vi "Verwaltung Betriebsstundenzaehler.vi"(8 "Zeitstempel Syslog":timestamp, 10 "Zeitstempel FT-IR":timestamp, 11 "Zeitstempel BMP":timestamp) -> (0 "Zeitstempel Syslog":timestamp, 2 "Zeitstempel FT-IR":timestamp, 3 "Zeitstempel BMP":timestamp)   [LabVIEW 2020, in "Betriebsstundenzaehler.lvlib"]
uses:
  Betriebsstundenzaehler.lvlib
  Allgemein/FGV Zustaende Aktionen.ctl
  FGV BSZ Aktionen.ctl
  Konfig-Dateien/Aktionen Konfig.ctl
  Regler/Druckregler/Aktionen Interne Werte.ctl
  SysLog/SysLog Interface cRIO.ctl
  Konfig-Dateien/Konfig-Dateien.lvlib
  Regler/Druckregler/Druckregler.lvlib
  Allgemein/Allgemein.lvlib
  SysLog/SysLog_cRIO.lvlib
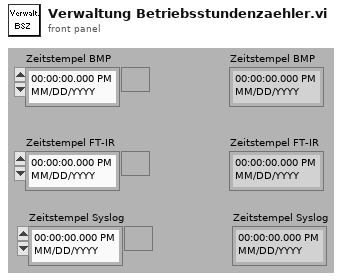
[diagram p1: front panel]
types:
  T1 = typedef "Allgemein.lvlib/FGV Zustaende Aktionen.ctl" = enum16{"lesen", "Zustand PC", "Zustand cRIO", "Bildnummer", "Samplepoint", "Sysloglevel"}
  T2 = typedef "Betriebsstundenzaehler.lvlib/FGV BSZ Aktionen.ctl" = enum16{"Lesen", "Initialisieren", "Starten Pumpe", "Zählen Pumpe", "Starten FT-IR", "Zählen FT-IR"}
  T3 = typedef "Regler.lvlib/Druckregler.lvlib/Aktionen Interne Werte.ctl" = enum16{"lesen", "FT-IR", "Ausgang", "Pumpe", "laden", "speichern", "Änderung?", "Druck Kalter Block", "Dichtheitstest"}
  T4 = typedef "Konfig-Dateien.lvlib/Aktionen Konfig.ctl" = enum16{"lesen", "laden", "speichern  System.ini", "speichern Anlagengrenzw.", "speichern PID + Sonstige", "speichern BSZ BMP", "speichern BSZ FT-IR", "speichern Stickstoff Bef.", "speichern Ext. Stickstoff Bef.", "speichern CAN_Konfig"}
  T5 = typedef "SysLog_cRIO.lvlib/SysLog Interface cRIO.ctl" = cluster{"FehlermeldungsCode":i32, "ErfolgsmeldungsCode":i32, "ParameterListenString":string, "intern":bool}
  T6 = typedef "Funktionstasten.lvlib/Zustaende.ctl" = enum16{"Standby", "Pause", "Eco", "Messen", "Kalibrieren", "Spülen Filter", "Spülen Leitung", "Umgebungsluft", "0-Gas", "Cal-Gas", "CG zu PNS", "-------------", "Init 1", "Init 2", "Init 3", "Init 4", "Messen vorbereiten", "Messen durchführen", "Exit"}
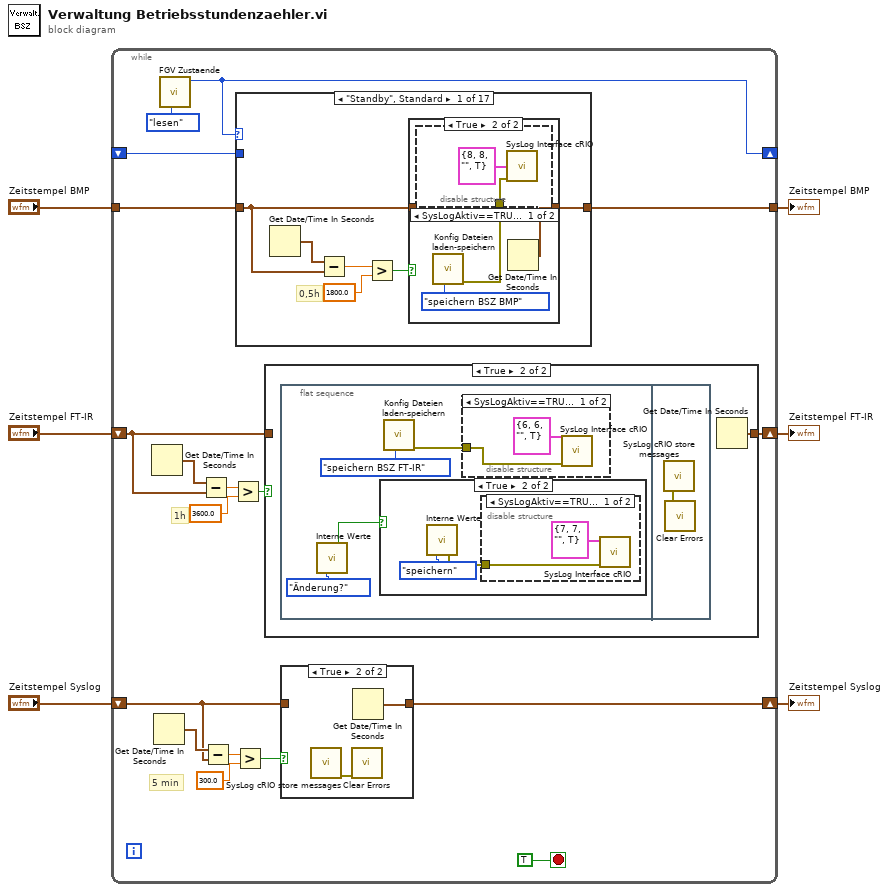
[diagram p0: block diagram]
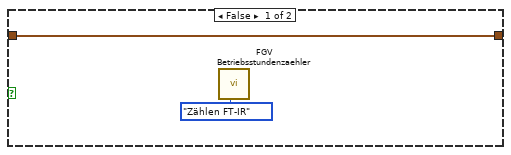
[diagram p3: hidden frame]
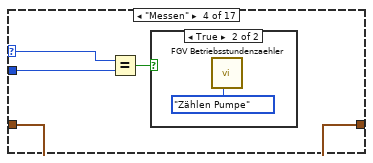
[diagram p11: hidden frame]
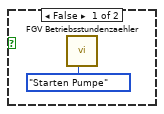
[diagram p12: hidden frame]
diagram:
  n1 = while {
    shift-right: [w13] -> _
    shift-left: _ -> [w23]
    tunnel: "Zeitstempel BMP" -> [w22]
    tunnel: [w21] -> w5
    shift-right: [w15] -> w3
    shift-left: "Zeitstempel FT-IR" -> [w16]
    shift-right: [w7] -> w1
    shift-left: "Zeitstempel Syslog" -> [w8]
    stop <- TRUE stop-if-true
    # "5 min"
    # "1h"
    n2 = Get Date/Time In Seconds() -> (seconds since 1Jan1904=w17:timestamp)
    n3 = Get Date/Time In Seconds() -> (seconds since 1Jan1904=w12:timestamp)
    n4 = call "FGV Zustaende.vi"("Aktionen"=FGV_Zustaende_Aktionen."lesen") -> ("Zustand PC"=w13:T6)  [unwired: 6 in, 4 out]
    n5 = Subtract(x=w17, y=w16) -> (x-y=w18:dbl)
    n6 = Subtract(x=w12, y=w8) -> (x-y=w11:dbl)
    n7 = Greater?(x=w18, y=3600.0) -> (0:w20:bool)
    n8 = Greater?(x=w11, y=300.0) -> (0:w9:bool)
    n9 = case shown="\"Standby\", Standard" w13 {
      selector: w13 -> [_ _ _ w58 _ _ _ _ _ _ _ _ _ _ _ _ _]
      tunnel: w23 -> [_ _ _ w57 _ _ _ _ _ _ _ _ _ _ _ _ _]
      tunnel: w22 -> [w42 w54 w55 w56 w62 w63 w64 w65 w66 w67 w68 w69 w70 w71 w72 w73 w74]
      tunnel: [w43 w54 w55 w56 w62 w63 w64 w65 w66 w67 w68 w69 w70 w71 w72 w73 w74] -> w21
      frame "Standby", Default {
        # "0,5h"
        n10 = Get Date/Time In Seconds() -> (seconds since 1Jan1904=w47:timestamp)
        n11 = Subtract(x=w47, y=w42) -> (x-y=w46:dbl)
        n12 = Greater?(x=w46, y=1800.0) -> (0:w44:bool)
        n13 = case shown="True" w44 {
          tunnel: [w48 w51] -> w43
          tunnel: w42 -> [w48 _]
          frame False {
          }
          frame True {
            n14 = call "Konfig Dateien laden-speichern.vi"("Aktion"=Aktionen_Konfig."speichern BSZ BMP") -> ("Fehler (Ausgang)"=w49:errorcluster)  [unwired: 10 in]
            n15 = disable-structure shown="SysLogAktiv==TRUE" {
              disable-tunnel: w49 -> [w53 _]
              frame condition #0 (active) {
                n16 = call "SysLog Interface cRIO.vi"("Fehler (in)"=w53, "Cluster (in)"=T5 {"FehlermeldungsCode"=8, "ErfolgsmeldungsCode"=8, "ParameterListenString"="", "intern"=TRUE}) -> ()  [unwired: 9 in, 1 out]
              }
              frame condition #1 {
              }
            }
            n17 = Get Date/Time In Seconds() -> (seconds since 1Jan1904=w51:timestamp)
          }
        }
      }
      frame "Pause" {
      }
      frame "Eco" {
      }
      frame "Messen" {
        n18 = Equal?(x=w58, y=w57) -> (x = y?=w59:bool)
        n19 = case shown="True" w59 {
          frame False {
            n20 = call "FGV Betriebsstundenzaehler.vi"("BSZ Aktionen"=FGV_BSZ_Aktionen."Starten Pumpe") -> ()  [unwired: 9 in, 2 out]
          }
          frame True {
            n21 = call "FGV Betriebsstundenzaehler.vi"("BSZ Aktionen"=FGV_BSZ_Aktionen."Zählen Pumpe") -> ()  [unwired: 9 in, 2 out]
          }
        }
      }
      frame "Kalibrieren" {
      }
      frame "Spülen Filter" {
      }
      frame "Spülen Leitung" {
      }
      frame "0-Gas" {
      }
      frame "Cal-Gas" {
      }
      frame "-------------" {
      }
      frame "Init 1" {
      }
      frame "Init 2" {
      }
      frame "Init 3" {
      }
      frame "Init 4" {
      }
      frame "Messen vorbereiten" {
      }
      frame "Messen durchführen" {
      }
      frame "Exit" {
      }
    }
    n22 = case shown="True" w20 {
      tunnel: [w28 w30] -> w15
      tunnel: w16 -> [w28 _]
      frame False {
        n23 = call "FGV Betriebsstundenzaehler.vi"("BSZ Aktionen"=FGV_BSZ_Aktionen."Zählen FT-IR") -> ()  [unwired: 9 in, 2 out]
      }
      frame True {
        n24 = flat-sequence {
          frame #0 {
            n25 = call "Interne Werte.vi"("Aktionen Interne Werte"=Aktionen_Interne_Werte."Änderung?") -> ("Änderung?"=w32:bool)  [unwired: 8 in, 6 out]
            n26 = case shown="True" w32 {
              frame False {
              }
              frame True {
                n27 = call "Interne Werte.vi"("Aktionen Interne Werte"=Aktionen_Interne_Werte."speichern") -> ("error out"=w37:errorcluster)  [unwired: 8 in, 6 out]
                n28 = disable-structure shown="SysLogAktiv==TRUE" {
                  disable-tunnel: w37 -> [w40 _]
                  frame condition #0 (active) {
                    n29 = call "SysLog Interface cRIO.vi"("Fehler (in)"=w40, "Cluster (in)"=T5 {"FehlermeldungsCode"=7, "ErfolgsmeldungsCode"=7, "ParameterListenString"="", "intern"=TRUE}) -> ()  [unwired: 9 in, 1 out]
                  }
                  frame condition #1 {
                  }
                }
              }
            }
            n30 = call "Konfig Dateien laden-speichern.vi"("Aktion"=Aktionen_Konfig."speichern BSZ FT-IR") -> ("Fehler (Ausgang)"=w31:errorcluster)  [unwired: 10 in]
            n31 = disable-structure shown="SysLogAktiv==TRUE" {
              disable-tunnel: w31 -> [w36 _]
              frame condition #0 (active) {
                n32 = call "SysLog Interface cRIO.vi"("Fehler (in)"=w36, "Cluster (in)"=T5 {"FehlermeldungsCode"=6, "ErfolgsmeldungsCode"=6, "ParameterListenString"="", "intern"=TRUE}) -> ()  [unwired: 9 in, 1 out]
              }
              frame condition #1 {
              }
            }
          }
          frame #1 {
            n33 = call "SysLog cRIO store messages.vi"() -> ("Fehler (out)"=w41:errorcluster)  [unwired: 11 in]
            n34 = call <vilib>:"Clear Errors.vi"("error in (no error)"=w41) -> ()  [unwired: 5 in, 2 out]
          }
        }
        n35 = Get Date/Time In Seconds() -> (seconds since 1Jan1904=w30:timestamp)
      }
    }
    n36 = case shown="True" w9 {
      tunnel: w8 -> [w25 _]
      tunnel: [w25 w26] -> w7
      frame False {
      }
      frame True {
        n37 = call "SysLog cRIO store messages.vi"() -> ("Fehler (out)"=w27:errorcluster)  [unwired: 11 in]
        n38 = call <vilib>:"Clear Errors.vi"("error in (no error)"=w27) -> ()  [unwired: 5 in, 2 out]
        n39 = Get Date/Time In Seconds() -> (seconds since 1Jan1904=w26:timestamp)
      }
    }
  }
  "Zeitstempel BMP" <- w5
  "Zeitstempel FT-IR" <- w3
  "Zeitstempel Syslog" <- w1
